vi "Write Hostname.vi"(8 "error in (no error)":errorcluster, 10 "Hostname":string, 11 "Test Suite in":refnum<class "Test Suite.lvclass">) -> (0 "error out":errorcluster, 3 "Test Suite out":refnum<class "Test Suite.lvclass">)   [LabVIEW 2013, in "JUnit XML.lvlib" / "Test Suite.lvclass"]
uses:
  Test Suite.lvclass
  Test Suite.lvclass/Test Suite.ctl
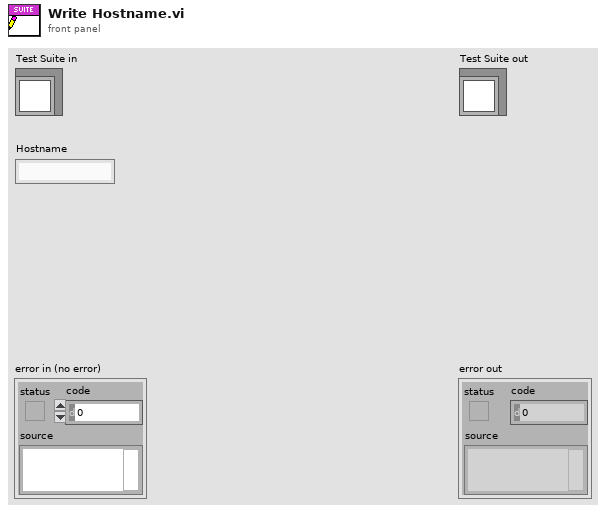
[diagram p1: front panel]
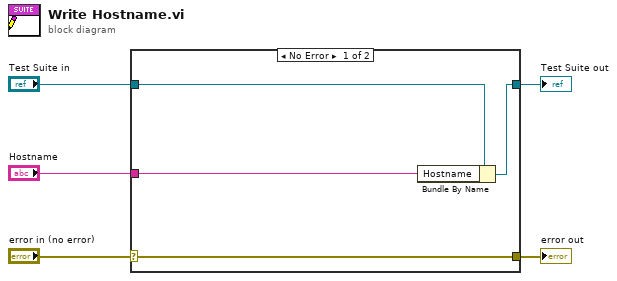
[diagram p0: block diagram]
diagram:
  n1 = case shown="No Error" "error in (no error)" {
    selector: "error in (no error)" -> [w9 w10]
    tunnel: [w9 w10] -> w4
    tunnel: [w7 w11] -> w2
    tunnel: "Test Suite in" -> [w8 w11]
    tunnel: "Hostname" -> [w6 _]
    frame No Error {
      n2 = Bundle By Name(cluster=w8, "Hostname"=w6) -> (w7:refnum<class "Test Suite.lvclass">)
    }
    frame Error {
    }
  }
  "error out" <- w4
  "Test Suite out" <- w2
